vi "Main -simul.vi"() -> ()   [LabVIEW 2013]
uses:
  <vilib>/userdefined/High Color/IMAQdx.ctl
  <vilib>/DAQmx/read.llb/DAQmx Read (Analog 1D Wfm NChan NSamp).vi
  <vilib>/Analysis/baseanly.llb/Mean (DBL).vi
  <vilib>/DAQmx/miscellaneous.llb/DAQmx Fill In Error Info.vi
  <vilib>/measure/madcrms.llb/Basic Averaged DC-RMS for 1 Chan.vi
  <vilib>/measure/mascope.llb/Amplitude and Levels 1 chan.vi
  <vilib>/measure/mamon.llb/Trigger Detection for 1 Channel.vi
  <vilib>/Waveform/WDTOps.llb/WDT Append Waveforms DBL.vi
  <vilib>/measure/NI_MAPro.lvlib
  <vilib>/Analysis/NI_AALBase.lvlib
  <vilib>/vision/driver/NI_Vision_Acquisition_Software.lvlib
panel:
  out "dt":u32
  in  "탭 컨트롤":T1(tab)
  out "웨이브폼 차트 2":dbl(graph)
  in  "reset":bool
  out "right":dbl(slide) scale=0.0..0.5
  out "left":dbl(slide)
  out "rear":dbl(slide) scale=0.0..0.5
  out "front":dbl(slide)
  out "trigger":bool
  in  "Force cal val":bool
  out "Triggered Force graph":waveform(dbl)(graph)={"t0"=timestamp(0 s since 1904-01-01), "dt"=0.00062, "Y"=array[3100 elements]}
  out "bonding force":dbl=1.1386680148675508 caption="Bonding force (kg)" format="%.3f"
  out "Bondtime":dbl=0.5053000000000001 caption="Bonding time" format="%.3f"
  out "vacum":dbl=1.2177873383633695 format="%#_3f"
  out "Heater temp":dbl=nan format="%0.2f"
  out "XY 그래프":cluster{dbl[], dbl[]}(graph)
  out "크기 2":i32[](array[numeric])
  out "triiger":bool
  out "숫자형":i32
  in  "simul":bool
  out "vaccum 차트 3":waveform(dbl)(graph)={"t0"=timestamp(3477442777.176875 s since 1904-01-01), "dt"=0.01, "Y"=[0.9261417940939543, 0.9261417940939543, 0.9261417940939543, 0.9261417940939543, 0.9261417940939543, 0.9261417940939543, 0.9261417940939543, 0.9261417940939543, 0.9261417940939543, 0.9261417940939543], "attributes"=variant("NI_ChannelName"=variant(string "전압"), "NI_UnitDescription"=variant(string "Volts"))}
  out "Force raw chart":waveform(dbl)[](graph)=[{"t0"=timestamp(3477442777.13187 s since 1904-01-01), "dt"=0.00062, "Y"=[-1.6112136636470233e-05, -8.569886798010926e-06, -1.9875060209823524e-07, 2.38297423695265e-06, -2.5658168581669667e-06, -1.772821098699811e-06, -4.127955201515539e-06, 6.359857628775875e-07, 4.928880013384412e-07, -3.030881455329775e-06, -1.6476111269731543e-06, -3.5257574105908386e-06, 3.9272455815972755e-06, 4.1657435117466915e-06, 1.9357923056845556e-06, -8.873963893666015e-06, -7.478785108954976e-06, 2.961286460921625e-07, 1.4110617831093333e-07, -1.8980310390713461e-06, 1.6734457588159683e-06, -1.091306434532689e-05, -1.0513727362142483e-06, -6.190924313818898e-06, -1.2540761368932031e-05, -2.1656959207560037e-05, -7.4907097304474685e-06, -3.2872630354662113e-06, -7.950263527933837e-08, -5.964355867846931e-06, -2.4107952296524134e-06, -3.7881010918357573e-06, 2.609546568115507e-06, 1.715182700246618e-06, -5.290612250873919e-06, -6.512889823589868e-06, -3.120361442334684e-07, 5.578846081749961e-06, 7.045614998740958e-06, -1.4627773018794912e-06, -7.937882831116044e-06, -2.595628704294203e-06, 1.2799261966089874e-06, 3.3190306855961753e-07, -3.4363220332503078e-06, -9.953137975658443e-06, 2.3591245238553327e-06, -1.0871470597100204e-06, 8.685197127258367e-07, -7.478785108954976e-06, -8.659321257106097e-06, -4.879210834785539e-06, -3.710590473067321e-06, -4.771888670569855e-06, -1.2516912366543758e-05, -5.576804340679935e-06, -6.274396873296863e-06, -8.546139112344271e-07, 2.2696881098723825e-06, -3.585380986597095e-06, -7.890184386099151e-06, 4.034519211733817e-07, 2.055040781583931e-06, 3.3071514956147953e-06, -2.7625750097582926e-06, -6.900440625190667e-06, 4.2909549706155075e-06, 9.830102788370948e-06, 3.032879356729265e-06, 4.088231671969834e-06, -9.488079817087242e-06, -5.111742111559042e-06, 2.567809552028929e-06, -4.688415860253707e-06, -1.833603522524735e-05, -9.50012139076079e-07, 3.3250388142463035e-06, -2.6135158111173114e-06, -6.769269618278701e-06, -2.0929577385222132e-05, -7.305878065355784e-06, -1.8562943957647073e-06, -3.090505090348801e-06, -3.5257574105908386e-06, -4.932871908254762e-06, -1.033522309183479e-07, -4.169691655199052e-06, 1.94771715199473e-06, -5.254838228130094e-06, -5.147516144541169e-06, 1.2978134427175586e-06, 9.126526251121246e-06, 1.5422725370008507e-06, -4.688415860253707e-06, -2.005353820147982e-06, 4.4518875659287035e-07, 1.7688444872052448e-06, -1.1229213806461855e-06, -6.51885214588969e-06, -1.4490413466475015e-05], "attributes"=variant("NI_ChannelName"=variant(string "변형률_0"), "NI_UnitDescription"=variant(string "Strain"))}, {"t0"=timestamp(3477442777.13187 s since 1904-01-01), "dt"=0.00062, "Y"=[-1.5926450874775857e-06, 1.7934307923881257e-06, -2.236473822173629e-06, -4.09045749208906e-06, -3.881810155491518e-06, 1.7218937409129746e-06, 3.9872386740088464e-06, 1.7192680555871353e-07, 2.2286147427125606e-06, -1.3005373326004466e-06, 3.456670124526979e-06, 8.523920832607e-06, 5.322604705970085e-06, 3.104945216654824e-06, 2.639953345335169e-06, 6.449322569493326e-06, 1.898110120282012e-07, -2.9306233811443237e-07, -7.929552945691535e-06, 2.53892933758521e-05, 6.6698972632327115e-06, 5.113953528386892e-06, 2.425341858268832e-06, -5.911320745626876e-07, -2.8385721664852527e-06, 1.0303694376600552e-06, -3.2286931975534613e-07, -4.793896442446842e-06, -2.7789585013682837e-06, -2.254357941858881e-06, 4.482039064584e-06, 3.188405341896096e-06, 2.890333530003795e-06, 1.5370897386411374e-06, 1.3224787249476363e-06, 5.0603003825103886e-06, 4.470116157849115e-06, 2.0378491288205883e-06, 3.087060905915481e-06, 4.237619533343155e-06, 6.22874797305966e-06, 2.4551490037417866e-06, 8.455656909807571e-07, -1.976799849226179e-07, -2.862417630541878e-06, 5.030493081733363e-06, 2.8068734545164028e-06, -7.640124402846258e-07, -2.105323591603382e-06, 2.3750223240719277e-07, 6.884510572159387e-06, -7.878580032793122e-07, -5.163499562134611e-06, -6.391533772034915e-06, -2.6835766223972933e-06, 4.684728522578421e-06, 2.885317683250044e-08, -1.2826531787987904e-06, -2.8206880676963555e-06, 3.7726266086577194e-06, 6.7414350226397595e-06, 3.3195569954219583e-06, 2.017338166964026e-07, 2.7114905281608864e-06, 3.40301715648635e-06, 9.60891530636603e-06, -7.029395011258529e-06, 2.153804825353152e-05, 1.1194680695472973e-05, -9.786224662971449e-07, 8.702765913475292e-06, -2.558387878634849e-06, -5.911320745626876e-07, -2.4272377325028147e-06, 2.8307191889483254e-06, 5.656446771208991e-06, 1.9901577367198323e-06, -2.2960875519699664e-06, -4.656785538247539e-06, -2.898185824494624e-06, 7.501831387741804e-07, -3.983153158427838e-06, -1.610529230191517e-06, -2.8028039682679484e-06, 4.458193251398366e-06, 9.171026170763248e-07, 3.748780829304955e-06, 1.9577241432685033e-07, 3.206289656260379e-06, 2.0974633753433343e-06, 7.442217298655735e-07, 6.548006047634227e-07, -1.8489844052503307e-06, 3.7964723891478954e-06, 8.0470009297029e-06, 2.5863004649327575e-06, 1.1674819390124968e-06, 3.150004752252312e-07, 3.188405341896096e-06, 5.7637531966593845e-06], "attributes"=variant("NI_ChannelName"=variant(string "변형률_1"), "NI_UnitDescription"=variant(string "Strain"))}, {"t0"=timestamp(3477442777.13187 s since 1904-01-01), "dt"=0.00062, "Y"=[-9.774144215970737e-06, -5.761376757146625e-06, 5.947220028941115e-07, -3.8056626676763385e-06, -7.275857412313684e-06, 3.1765375395588494e-06, -3.1557437920494864e-06, -3.000717146469372e-06, 7.974506851273759e-07, -1.8618660842482212e-06, -1.4862235419361472e-06, -6.721343374039278e-06, 8.62045556081355e-06, -3.294812422418737e-07, 2.115189123215763e-06, -2.3030966465335333e-06, -5.773301819593379e-06, -1.1940569250260916e-06, -5.171085810533189e-06, -2.538875015539028e-08, 3.6814298472928053e-07, -8.939395837287375e-06, 2.401395215885246e-06, -4.646382161832467e-06, -7.311632490439199e-06, -2.205074690463858e-05, -3.5313850800753163e-06, -4.425767963291082e-06, -3.6148608835335274e-06, -1.677026138378287e-06, -2.5952626153941553e-06, 3.26404755740087e-07, -2.601225184409818e-06, 1.4056372250135049e-06, -1.1753684800069817e-05, -4.914696596438629e-06, 5.808765257422834e-08, 6.318857576908811e-06, 3.9934195965366175e-06, 5.03688401927312e-06, -6.059503232998047e-06, -5.4811377077647035e-06, 1.3937119916306282e-06, -7.055244373975443e-06, 7.318619848217363e-07, -1.718764196644247e-06, 4.814324809771893e-07, -1.0119968136008337e-05, 1.984011385493666e-06, -1.0131893094502119e-05, -1.0251142663796572e-05, -3.865288210289022e-06, -6.06546576070178e-06, -6.995619211769368e-06, 2.1867406310243084e-06, -1.0119968136008337e-05, -8.080796051007461e-06, -1.7962777241804084e-06, -1.2536827790775241e-06, 1.4771886312832808e-06, 2.2284790153078483e-06, -6.190678826058288e-06, -1.7068390374955085e-06, 1.4593007787556523e-06, 5.024958699283277e-06, 2.1927032571370627e-06, 5.589463616211063e-07, -4.831221009990731e-06, -8.959275481128778e-07, 3.421005752440379e-06, 3.987456948949547e-06, -4.205153667407975e-06, -9.674786147839707e-07, -5.212823577128643e-06, -1.6183772832057885e-05, 9.294241431321112e-06, -3.257107342016943e-06, -4.473468338791205e-06, -1.0316729914785664e-05, -1.128265025116678e-05, -1.0650628513704086e-05, -4.65234470638786e-06, -2.362722368329657e-06, -7.230124280525015e-07, 7.139741589589915e-07, -2.326946936105031e-06, -1.5277486145651072e-05, 1.411599841811428e-06, -3.3703959911923048e-06, -5.7852268817560655e-06, 2.17481537901177e-06, 2.5325730631100896e-06, -1.981117625965015e-06, -2.3209843638189005e-06, -2.6191128910294843e-06, 9.047776678219688e-07, -6.514613263977364e-07, -9.495908490762017e-07, 5.470211484321648e-07, -1.2970025127066287e-05], "attributes"=variant("NI_ChannelName"=variant(string "변형률_2"), "NI_UnitDescription"=variant(string "Strain"))}, {"t0"=timestamp(3477442777.13187 s since 1904-01-01), "dt"=0.00062, "Y"=[-7.598292136517871e-06, -3.990960943167142e-06, -3.961148180242939e-06, 8.446924425047726e-07, -3.865747326939833e-06, -6.459578537381319e-07, -5.028556181360945e-07, -4.313044849763774e-07, -2.0352399287900154e-06, -2.1843042998043006e-06, 2.317459299605134e-06, 2.520188680335006e-06, 1.8642998046072807e-06, 3.1998303138911986e-07, -2.3810692014959805e-06, 1.1129194138591358e-07, -3.919410309162601e-06, -4.181762583788524e-06, -2.9177003579997263e-06, -2.887887531081505e-06, 8.147893563887326e-08, -5.910899132064934e-06, 5.841384650575335e-06, -7.771348670609545e-07, -9.965402760758176e-06, -5.064219224553743e-06, -1.0078689889986319e-05, -8.14684269941332e-06, -4.8913055460130025e-06, -2.0292773530250545e-06, -2.5003206193811262e-06, -4.098286874975869e-06, -3.305266946174274e-06, -4.038661360148547e-06, -2.4228072009909966e-06, -2.1366037059148034e-06, -4.217537883299131e-06, -1.2183663865814867e-06, -2.5062831895288145e-06, 1.1725454274867201e-07, 3.9571845882479464e-06, -1.8087543828407676e-07, -4.0803992212742764e-06, -1.2064412154978175e-06, -5.839348772806825e-06, -1.8563626249113895e-06, -5.213282692541838e-06, -3.1800531582297593e-06, -1.8742503581789873e-06, -3.8360372384809986e-07, -4.181762583788524e-06, -6.0420747641119605e-06, -4.050586463682811e-06, -3.531844197032469e-06, -2.3452937705841765e-06, -7.1034036122986465e-06, -1.32569291353597e-06, -1.6953729967054738e-06, -1.7549987909737935e-06, -2.8699998340773e-06, -4.825717583337447e-06, -2.46454519700197e-06, 1.1964865605783791e-06, 3.378708431566748e-07, 2.889871880335409e-06, 2.0908795007679327e-06, -1.0514139655274806e-06, 5.501512595474361e-06, -3.376817668063878e-06, -4.819755040849376e-06, -1.5701588055974375e-06, -5.064219224553743e-06, -8.904240781442745e-07, 4.028736359651292e-06, -4.1996502338637966e-06, -6.918565604118794e-06, -3.996923495538705e-06, -3.3648925484600175e-06, -1.3024146240405366e-05, -8.289942747279497e-06, -7.061666003521132e-06, -5.165582387620764e-06, -6.823165315097408e-06, -1.0633391403086943e-06, -1.9517638616103747e-06, -5.255020455614867e-06, -2.4705077675762867e-06, -1.7491284040547266e-07, -3.1919782822420984e-06, -2.858074702385669e-06, -1.9815767443457687e-06, 2.317459299605134e-06, 3.927371353185168e-06, 3.665014961285459e-06, 2.186281508816372e-06, -1.0096758515535991e-06, -1.5522710614508004e-06, -6.507151727700881e-06, -2.16045400342839e-06, -2.893850096607393e-06], "attributes"=variant("NI_ChannelName"=variant(string "변형률_3"), "NI_UnitDescription"=variant(string "Strain"))}]
  in  "display":bool=TRUE
  out "vacum 2":dbl=0.9261417940939543 format="%#_3f"
  out "x-y 2":u32=56
  out "x-y":u32=99
  out "Filtered force 차트":waveform(dbl)[](graph)
  out "Force raw graph":waveform(dbl)[](graph)=[{"t0"=timestamp(3477442777.13187 s since 1904-01-01), "dt"=0.00062, "Y"=[-1.6112136636470233e-05, -8.569886798010926e-06, -1.9875060209823524e-07, 2.38297423695265e-06, -2.5658168581669667e-06, -1.772821098699811e-06, -4.127955201515539e-06, 6.359857628775875e-07, 4.928880013384412e-07, -3.030881455329775e-06, -1.6476111269731543e-06, -3.5257574105908386e-06, 3.9272455815972755e-06, 4.1657435117466915e-06, 1.9357923056845556e-06, -8.873963893666015e-06, -7.478785108954976e-06, 2.961286460921625e-07, 1.4110617831093333e-07, -1.8980310390713461e-06, 1.6734457588159683e-06, -1.091306434532689e-05, -1.0513727362142483e-06, -6.190924313818898e-06, -1.2540761368932031e-05, -2.1656959207560037e-05, -7.4907097304474685e-06, -3.2872630354662113e-06, -7.950263527933837e-08, -5.964355867846931e-06, -2.4107952296524134e-06, -3.7881010918357573e-06, 2.609546568115507e-06, 1.715182700246618e-06, -5.290612250873919e-06, -6.512889823589868e-06, -3.120361442334684e-07, 5.578846081749961e-06, 7.045614998740958e-06, -1.4627773018794912e-06, -7.937882831116044e-06, -2.595628704294203e-06, 1.2799261966089874e-06, 3.3190306855961753e-07, -3.4363220332503078e-06, -9.953137975658443e-06, 2.3591245238553327e-06, -1.0871470597100204e-06, 8.685197127258367e-07, -7.478785108954976e-06, -8.659321257106097e-06, -4.879210834785539e-06, -3.710590473067321e-06, -4.771888670569855e-06, -1.2516912366543758e-05, -5.576804340679935e-06, -6.274396873296863e-06, -8.546139112344271e-07, 2.2696881098723825e-06, -3.585380986597095e-06, -7.890184386099151e-06, 4.034519211733817e-07, 2.055040781583931e-06, 3.3071514956147953e-06, -2.7625750097582926e-06, -6.900440625190667e-06, 4.2909549706155075e-06, 9.830102788370948e-06, 3.032879356729265e-06, 4.088231671969834e-06, -9.488079817087242e-06, -5.111742111559042e-06, 2.567809552028929e-06, -4.688415860253707e-06, -1.833603522524735e-05, -9.50012139076079e-07, 3.3250388142463035e-06, -2.6135158111173114e-06, -6.769269618278701e-06, -2.0929577385222132e-05, -7.305878065355784e-06, -1.8562943957647073e-06, -3.090505090348801e-06, -3.5257574105908386e-06, -4.932871908254762e-06, -1.033522309183479e-07, -4.169691655199052e-06, 1.94771715199473e-06, -5.254838228130094e-06, -5.147516144541169e-06, 1.2978134427175586e-06, 9.126526251121246e-06, 1.5422725370008507e-06, -4.688415860253707e-06, -2.005353820147982e-06, 4.4518875659287035e-07, 1.7688444872052448e-06, -1.1229213806461855e-06, -6.51885214588969e-06, -1.4490413466475015e-05], "attributes"=variant("NI_ChannelName"=variant(string "변형률_0"), "NI_UnitDescription"=variant(string "Strain"))}, {"t0"=timestamp(3477442777.13187 s since 1904-01-01), "dt"=0.00062, "Y"=[-1.5926450874775857e-06, 1.7934307923881257e-06, -2.236473822173629e-06, -4.09045749208906e-06, -3.881810155491518e-06, 1.7218937409129746e-06, 3.9872386740088464e-06, 1.7192680555871353e-07, 2.2286147427125606e-06, -1.3005373326004466e-06, 3.456670124526979e-06, 8.523920832607e-06, 5.322604705970085e-06, 3.104945216654824e-06, 2.639953345335169e-06, 6.449322569493326e-06, 1.898110120282012e-07, -2.9306233811443237e-07, -7.929552945691535e-06, 2.53892933758521e-05, 6.6698972632327115e-06, 5.113953528386892e-06, 2.425341858268832e-06, -5.911320745626876e-07, -2.8385721664852527e-06, 1.0303694376600552e-06, -3.2286931975534613e-07, -4.793896442446842e-06, -2.7789585013682837e-06, -2.254357941858881e-06, 4.482039064584e-06, 3.188405341896096e-06, 2.890333530003795e-06, 1.5370897386411374e-06, 1.3224787249476363e-06, 5.0603003825103886e-06, 4.470116157849115e-06, 2.0378491288205883e-06, 3.087060905915481e-06, 4.237619533343155e-06, 6.22874797305966e-06, 2.4551490037417866e-06, 8.455656909807571e-07, -1.976799849226179e-07, -2.862417630541878e-06, 5.030493081733363e-06, 2.8068734545164028e-06, -7.640124402846258e-07, -2.105323591603382e-06, 2.3750223240719277e-07, 6.884510572159387e-06, -7.878580032793122e-07, -5.163499562134611e-06, -6.391533772034915e-06, -2.6835766223972933e-06, 4.684728522578421e-06, 2.885317683250044e-08, -1.2826531787987904e-06, -2.8206880676963555e-06, 3.7726266086577194e-06, 6.7414350226397595e-06, 3.3195569954219583e-06, 2.017338166964026e-07, 2.7114905281608864e-06, 3.40301715648635e-06, 9.60891530636603e-06, -7.029395011258529e-06, 2.153804825353152e-05, 1.1194680695472973e-05, -9.786224662971449e-07, 8.702765913475292e-06, -2.558387878634849e-06, -5.911320745626876e-07, -2.4272377325028147e-06, 2.8307191889483254e-06, 5.656446771208991e-06, 1.9901577367198323e-06, -2.2960875519699664e-06, -4.656785538247539e-06, -2.898185824494624e-06, 7.501831387741804e-07, -3.983153158427838e-06, -1.610529230191517e-06, -2.8028039682679484e-06, 4.458193251398366e-06, 9.171026170763248e-07, 3.748780829304955e-06, 1.9577241432685033e-07, 3.206289656260379e-06, 2.0974633753433343e-06, 7.442217298655735e-07, 6.548006047634227e-07, -1.8489844052503307e-06, 3.7964723891478954e-06, 8.0470009297029e-06, 2.5863004649327575e-06, 1.1674819390124968e-06, 3.150004752252312e-07, 3.188405341896096e-06, 5.7637531966593845e-06], "attributes"=variant("NI_ChannelName"=variant(string "변형률_1"), "NI_UnitDescription"=variant(string "Strain"))}, {"t0"=timestamp(3477442777.13187 s since 1904-01-01), "dt"=0.00062, "Y"=[-9.774144215970737e-06, -5.761376757146625e-06, 5.947220028941115e-07, -3.8056626676763385e-06, -7.275857412313684e-06, 3.1765375395588494e-06, -3.1557437920494864e-06, -3.000717146469372e-06, 7.974506851273759e-07, -1.8618660842482212e-06, -1.4862235419361472e-06, -6.721343374039278e-06, 8.62045556081355e-06, -3.294812422418737e-07, 2.115189123215763e-06, -2.3030966465335333e-06, -5.773301819593379e-06, -1.1940569250260916e-06, -5.171085810533189e-06, -2.538875015539028e-08, 3.6814298472928053e-07, -8.939395837287375e-06, 2.401395215885246e-06, -4.646382161832467e-06, -7.311632490439199e-06, -2.205074690463858e-05, -3.5313850800753163e-06, -4.425767963291082e-06, -3.6148608835335274e-06, -1.677026138378287e-06, -2.5952626153941553e-06, 3.26404755740087e-07, -2.601225184409818e-06, 1.4056372250135049e-06, -1.1753684800069817e-05, -4.914696596438629e-06, 5.808765257422834e-08, 6.318857576908811e-06, 3.9934195965366175e-06, 5.03688401927312e-06, -6.059503232998047e-06, -5.4811377077647035e-06, 1.3937119916306282e-06, -7.055244373975443e-06, 7.318619848217363e-07, -1.718764196644247e-06, 4.814324809771893e-07, -1.0119968136008337e-05, 1.984011385493666e-06, -1.0131893094502119e-05, -1.0251142663796572e-05, -3.865288210289022e-06, -6.06546576070178e-06, -6.995619211769368e-06, 2.1867406310243084e-06, -1.0119968136008337e-05, -8.080796051007461e-06, -1.7962777241804084e-06, -1.2536827790775241e-06, 1.4771886312832808e-06, 2.2284790153078483e-06, -6.190678826058288e-06, -1.7068390374955085e-06, 1.4593007787556523e-06, 5.024958699283277e-06, 2.1927032571370627e-06, 5.589463616211063e-07, -4.831221009990731e-06, -8.959275481128778e-07, 3.421005752440379e-06, 3.987456948949547e-06, -4.205153667407975e-06, -9.674786147839707e-07, -5.212823577128643e-06, -1.6183772832057885e-05, 9.294241431321112e-06, -3.257107342016943e-06, -4.473468338791205e-06, -1.0316729914785664e-05, -1.128265025116678e-05, -1.0650628513704086e-05, -4.65234470638786e-06, -2.362722368329657e-06, -7.230124280525015e-07, 7.139741589589915e-07, -2.326946936105031e-06, -1.5277486145651072e-05, 1.411599841811428e-06, -3.3703959911923048e-06, -5.7852268817560655e-06, 2.17481537901177e-06, 2.5325730631100896e-06, -1.981117625965015e-06, -2.3209843638189005e-06, -2.6191128910294843e-06, 9.047776678219688e-07, -6.514613263977364e-07, -9.495908490762017e-07, 5.470211484321648e-07, -1.2970025127066287e-05], "attributes"=variant("NI_ChannelName"=variant(string "변형률_2"), "NI_UnitDescription"=variant(string "Strain"))}, {"t0"=timestamp(3477442777.13187 s since 1904-01-01), "dt"=0.00062, "Y"=[-7.598292136517871e-06, -3.990960943167142e-06, -3.961148180242939e-06, 8.446924425047726e-07, -3.865747326939833e-06, -6.459578537381319e-07, -5.028556181360945e-07, -4.313044849763774e-07, -2.0352399287900154e-06, -2.1843042998043006e-06, 2.317459299605134e-06, 2.520188680335006e-06, 1.8642998046072807e-06, 3.1998303138911986e-07, -2.3810692014959805e-06, 1.1129194138591358e-07, -3.919410309162601e-06, -4.181762583788524e-06, -2.9177003579997263e-06, -2.887887531081505e-06, 8.147893563887326e-08, -5.910899132064934e-06, 5.841384650575335e-06, -7.771348670609545e-07, -9.965402760758176e-06, -5.064219224553743e-06, -1.0078689889986319e-05, -8.14684269941332e-06, -4.8913055460130025e-06, -2.0292773530250545e-06, -2.5003206193811262e-06, -4.098286874975869e-06, -3.305266946174274e-06, -4.038661360148547e-06, -2.4228072009909966e-06, -2.1366037059148034e-06, -4.217537883299131e-06, -1.2183663865814867e-06, -2.5062831895288145e-06, 1.1725454274867201e-07, 3.9571845882479464e-06, -1.8087543828407676e-07, -4.0803992212742764e-06, -1.2064412154978175e-06, -5.839348772806825e-06, -1.8563626249113895e-06, -5.213282692541838e-06, -3.1800531582297593e-06, -1.8742503581789873e-06, -3.8360372384809986e-07, -4.181762583788524e-06, -6.0420747641119605e-06, -4.050586463682811e-06, -3.531844197032469e-06, -2.3452937705841765e-06, -7.1034036122986465e-06, -1.32569291353597e-06, -1.6953729967054738e-06, -1.7549987909737935e-06, -2.8699998340773e-06, -4.825717583337447e-06, -2.46454519700197e-06, 1.1964865605783791e-06, 3.378708431566748e-07, 2.889871880335409e-06, 2.0908795007679327e-06, -1.0514139655274806e-06, 5.501512595474361e-06, -3.376817668063878e-06, -4.819755040849376e-06, -1.5701588055974375e-06, -5.064219224553743e-06, -8.904240781442745e-07, 4.028736359651292e-06, -4.1996502338637966e-06, -6.918565604118794e-06, -3.996923495538705e-06, -3.3648925484600175e-06, -1.3024146240405366e-05, -8.289942747279497e-06, -7.061666003521132e-06, -5.165582387620764e-06, -6.823165315097408e-06, -1.0633391403086943e-06, -1.9517638616103747e-06, -5.255020455614867e-06, -2.4705077675762867e-06, -1.7491284040547266e-07, -3.1919782822420984e-06, -2.858074702385669e-06, -1.9815767443457687e-06, 2.317459299605134e-06, 3.927371353185168e-06, 3.665014961285459e-06, 2.186281508816372e-06, -1.0096758515535991e-06, -1.5522710614508004e-06, -6.507151727700881e-06, -2.16045400342839e-06, -2.893850096607393e-06], "attributes"=variant("NI_ChannelName"=variant(string "변형률_3"), "NI_UnitDescription"=variant(string "Strain"))}]
  out "Filtered force 그래프":waveform(dbl)[](graph)
  out "Strain front":dbl(graph)=0.21080623907694704
  out "Strain left":dbl(graph)=0.40238302318753916
  out "Strain rear":dbl(graph)=0.4140902820131476
  out "Strain right":dbl(graph)=0.09497703213784708
  out "강도 그래프 2":dbl[][](graph)=[[nan, nan, nan, nan], [nan, nan, nan, nan]]
  out "Image":T2(plugin-control)
  out "error out":errorcluster={"status"=FALSE, "code"=-1074360308, "source"=""}
  out "Heater temp 2":dbl=nan caption="Heater temp" format="%0.2f"
  out "웨이브폼 차트":u32(graph)
  out "data":dynamicdata(graph)=[{"t0"=timestamp(3477442777.176875 s since 1904-01-01), "dt"=0.01, "Y"=[0.9261417940939543, 0.9261417940939543, 0.9261417940939543, 0.9261417940939543, 0.9261417940939543, 0.9261417940939543, 0.9261417940939543, 0.9261417940939543, 0.9261417940939543, 0.9261417940939543], "attributes"=variant("NI_ChannelName"=variant(string "전압"), "NI_UnitDescription"=variant(string "Volts"))}] caption="데이터"
  in  "bonding time trigger edge level":dbl=0.5 format="%#_13g"
  out "front mean":dbl=0.24100886710135544 format="%0.2f"
  out "left mean":dbl=0.5329196805184643 format="%0.2f"
  out "rear mean 3":dbl=0.3563222576715275 caption="rear mean" format="%0.2f"
  out "right mean 4":dbl=0.1826222935697912 caption="right mean" format="%0.2f"
  in  "Force trigger minimum level":dbl=0.5 format="%#_13g"
  in  "state settings":T3={"method"=enum."histogram", "histogram size"=512, "histogram method"=enum."mode", "reserved"=1.0} caption="상태 셋팅" {"reserved" format="%0.2f"}
  out "level1 4":dbl=0.09497703213784708 caption="right F" format="%.2g"
  out "level1 3":dbl=0.4140902820131476 caption="rear F" format="%.2g"
  out "level1 2":dbl=0.40238302318753916 caption="left F" format="%.2g"
  out "level1":dbl=0.21080623907694704 caption="front F" format="%.2g"
  in  "Lower Cut-Off":dbl=20.0 caption="하위 컷오프"
  out "웨이브폼 그래프 2":waveform(dbl)(graph)
  out "웨이브폼 그래프":waveform(dbl)(graph)
  out "force offset":dbl
  out "trigger location 2":dbl=1.84016 caption="트리거 falling" format="%#.3f"
  out "trigger location":dbl=1.33486 caption="트리거 rising" format="%#.3f"
  out "strain high level mean":T4={"mean"=0.24100886710135544, "mean"=0.5329196805184643, "mean"=0.3563222576715275, "mean"=0.1826222935697912}
  in  "정지":bool=TRUE
  # "Die Attach Machine Monitoring"
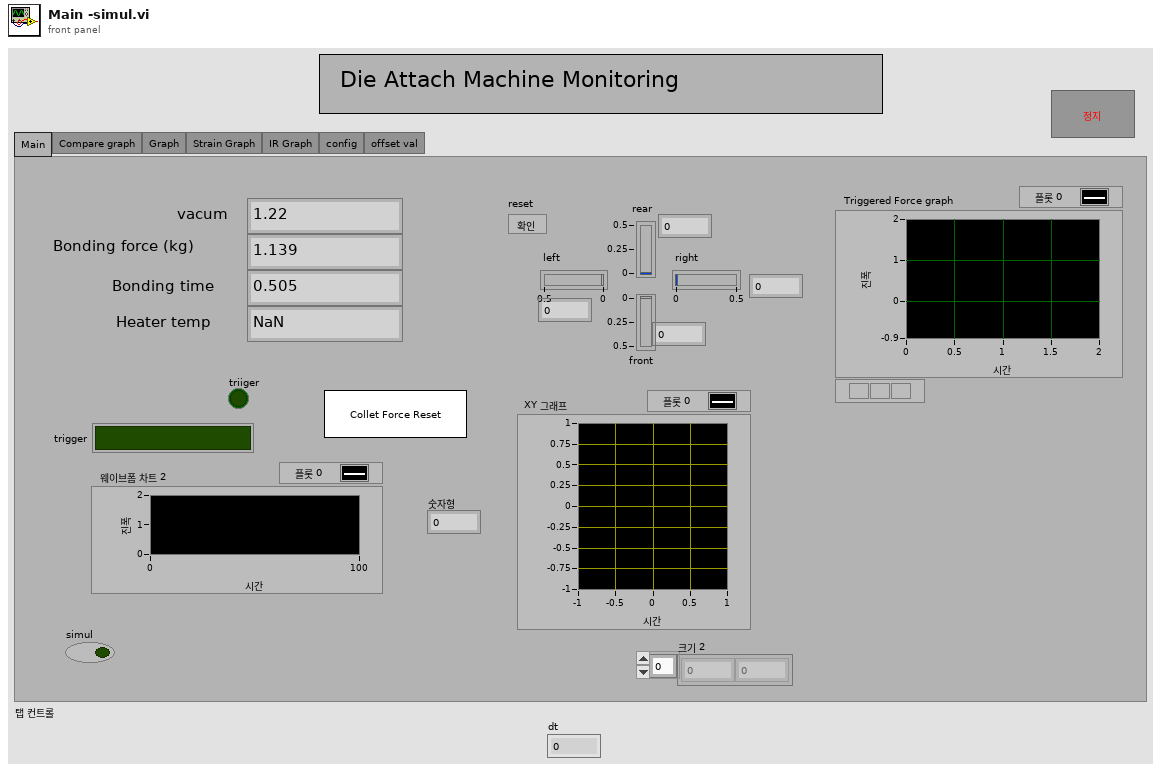
[diagram p1: front panel]
types:
  T1 = enum32{"Main", "Compare graph", "Graph", "Strain Graph", "IR Graph", "config", "offset val"}
  T2 = typedef "IMAQ Image.ctl" = refnum<image>
  T3 = cluster{"method":enum32{"histogram", "peak", "auto select"}, "histogram size":i32, "histogram method":enum16{"mode"}, "reserved":dbl}
  T4 = cluster{"mean":dbl, "mean":dbl, "mean":dbl, "mean":dbl}
  T5 = typedef "IMAQdx.ctl" = refnum<k21>
  T6 = cluster{"Global Rectangle":i32[], "Contours":cluster{"Contour Type":u32, "ROI Type":u32, "Points":i32[]}[]}
  T7 = cluster{"high state level":dbl, "high state level":dbl, "high state level":dbl, "high state level":dbl}
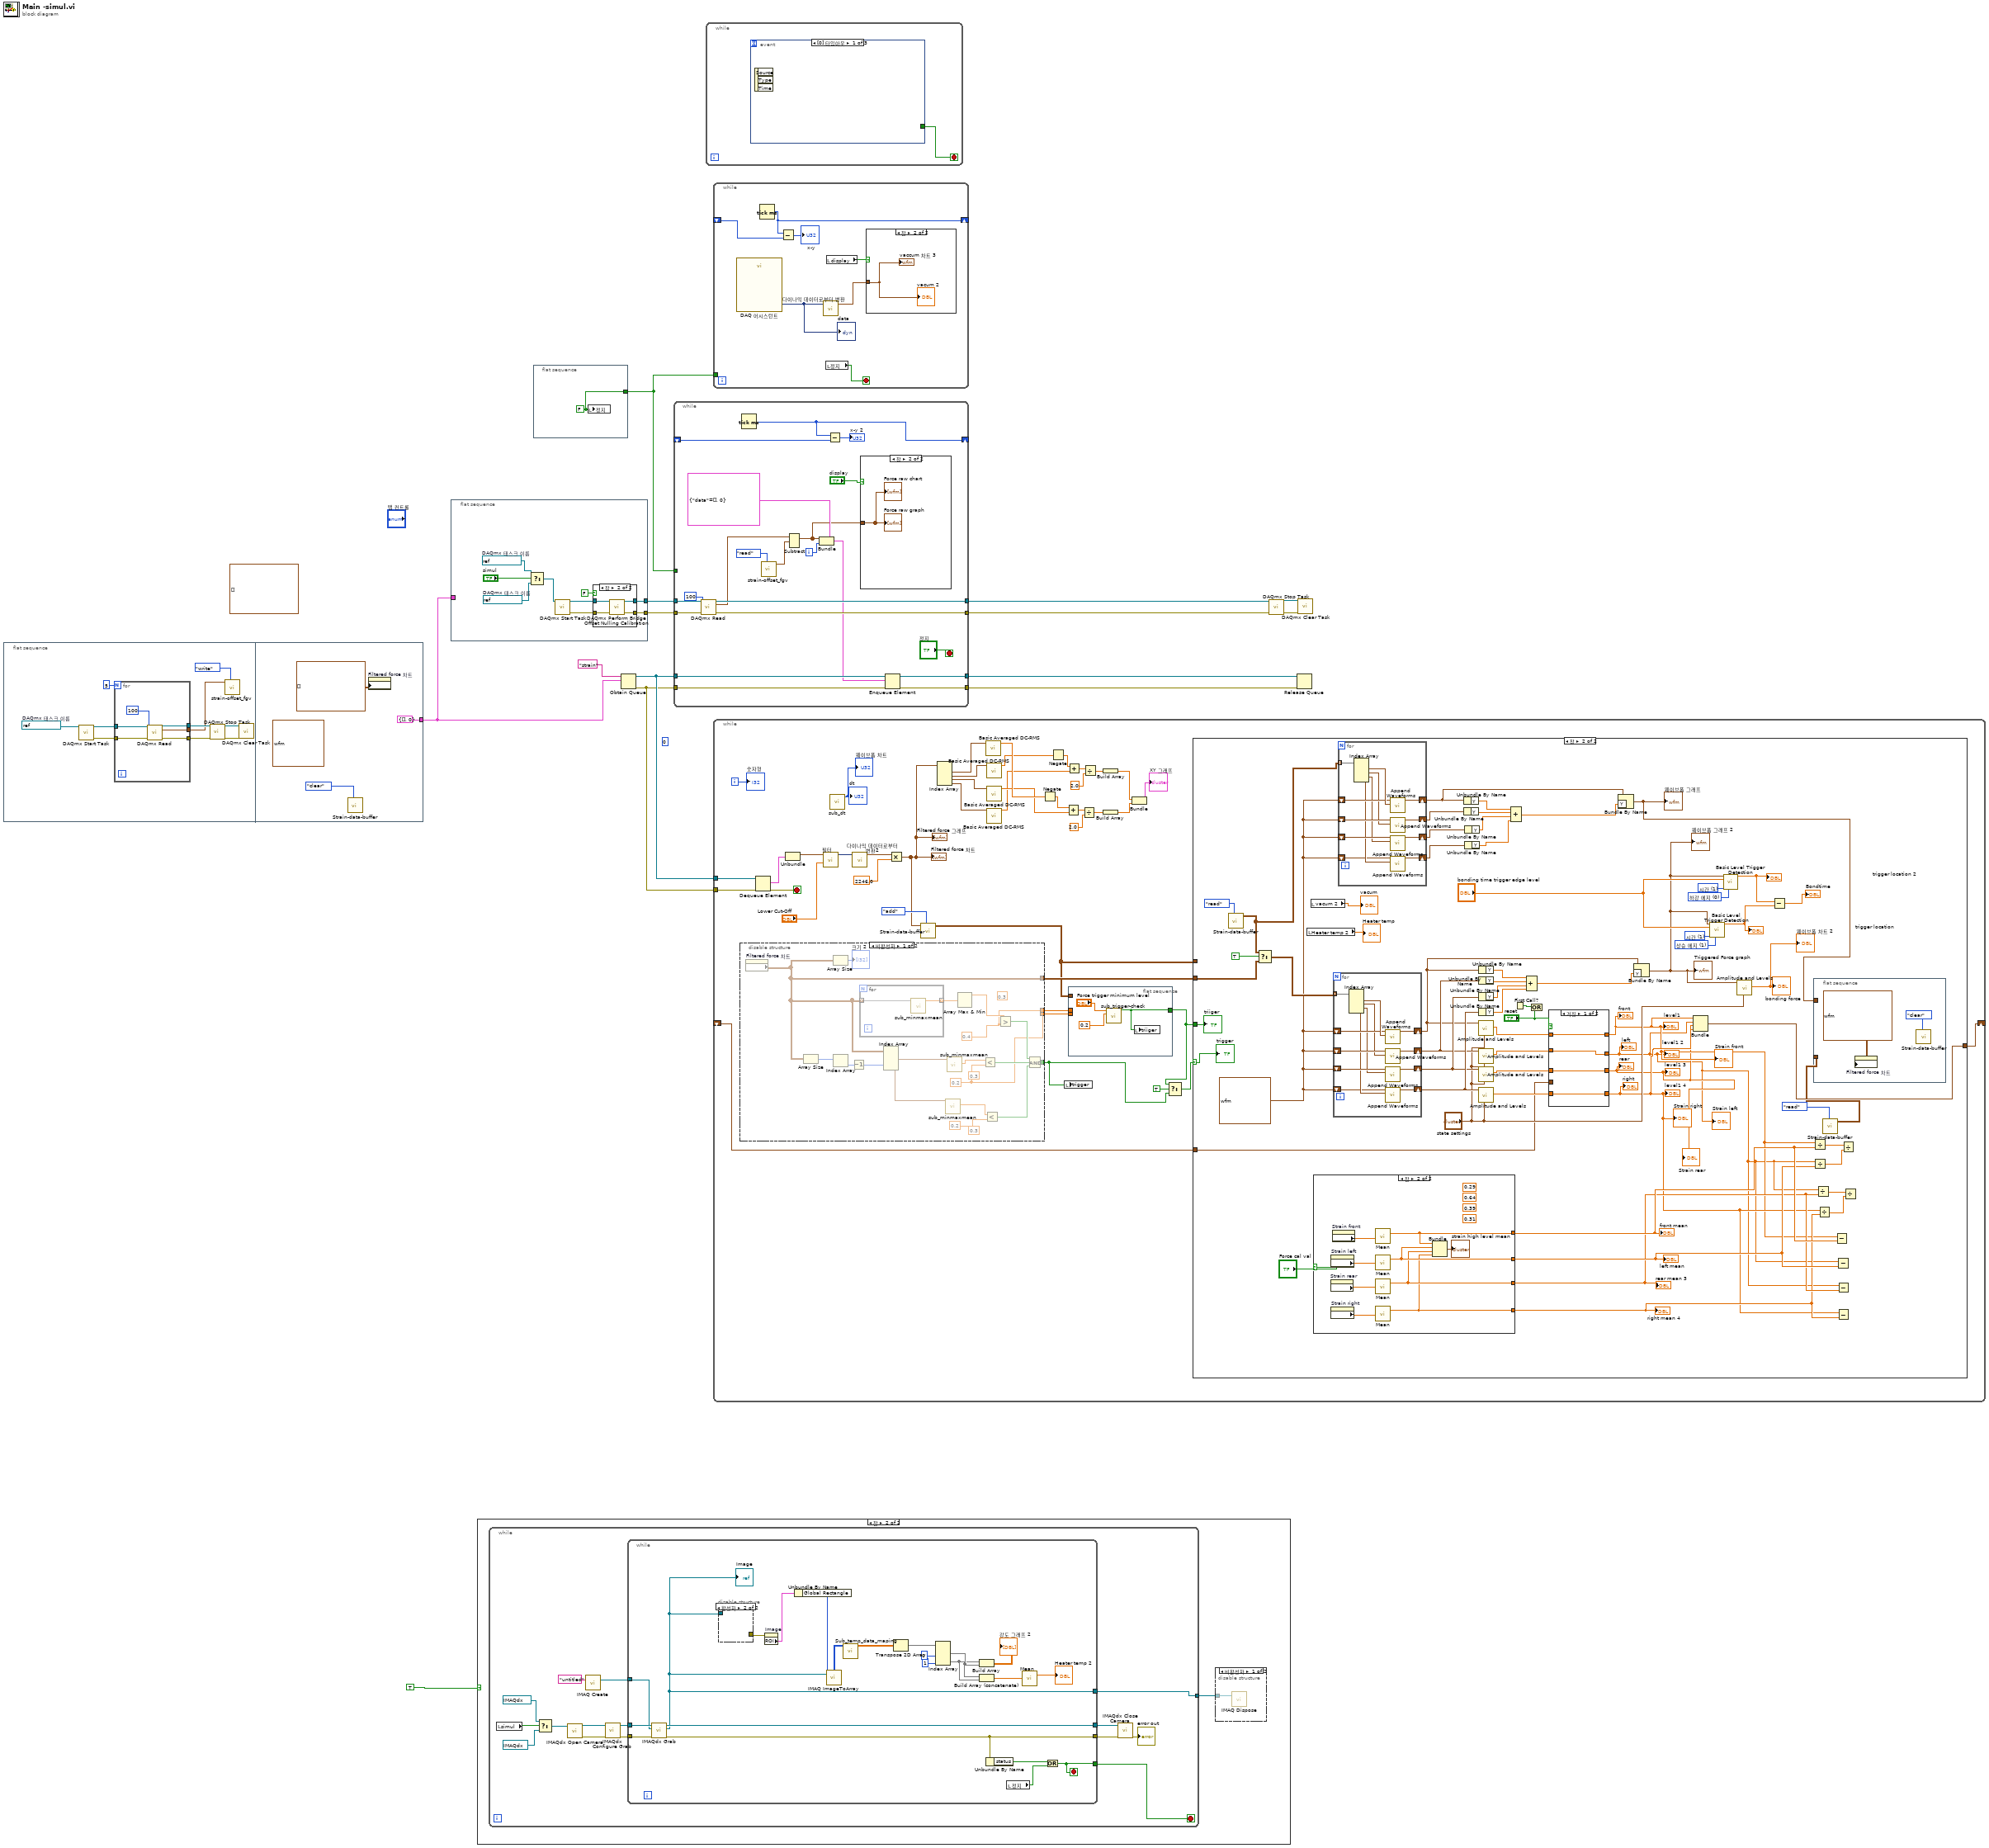
[diagram p0: block diagram]
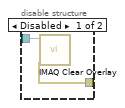
[diagram p4: hidden frame]
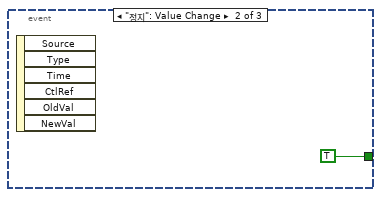
[diagram p6: hidden frame]
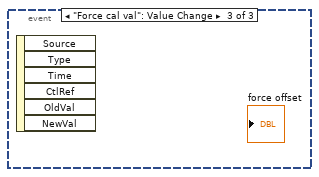
[diagram p7: hidden frame]
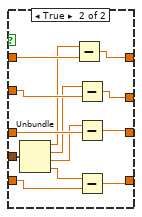
[diagram p10: hidden frame]
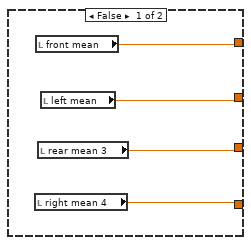
[diagram p11: hidden frame]
diagram:
  (unwired) waveform(dbl)[] [] ("data")
  (unwired) 0 ("y")
  n1 = flat-sequence {
    tunnel: [cluster{"data":waveform(dbl)[], i32} {"data"=[], 0}] -> w1
    frame #0 {
      w24 = refnum<k21> "9237_task"  # DAQmx 태스크 이름
      n2 = call <vilib>:"DAQmx Start Task.vi"("task/channels in"=w24) -> ("task out"=w22:refnum<k21>, "error out"=w23:errorcluster)  [unwired: 13 in]
      n3 = for {
        N: 5 -> [_]
        tunnel: w23 -> [w29]
        tunnel: w22 -> [w28]
        tunnel: [w27] -> w19
        tunnel: [w26] -> w18
        tunnel: [w25] -> w16
        n4 = call-poly <vilib>:"DAQmx Read.vi"("task/channels in"=w28, "number of samples per channel"=100, "error in"=w29) -> ("task out"=w26:refnum<k21>, "data"=w25:waveform(dbl)[], "error out"=w27:errorcluster)  [unwired: 10 in]
      }
      n5 = call <vilib>:"DAQmx Stop Task.vi"("task/channels in"=w18, "error in"=w19) -> ("task out"=w20:refnum<k21>, "error out"=w21:errorcluster)  [unwired: 12 in]
      n6 = call "strain-offset_fgv.vi"("열거형"=enum16{"write", "read"}."write", "data"=w16) -> ()  [unwired: 9 in, 1 out]
      n7 = call <vilib>:"DAQmx Clear Task.vi"("task in"=w20, "error in"=w21) -> ()  [unwired: 13 in, 1 out]
    }
    frame #1 {
      (unwired) waveform(dbl) {"t0"=timestamp(0 s since 1904-01-01), "dt"=1.0, "Y"=[]} ("Waveform")
      n8 = call "Strain-data-buffer.vi"("cmd"=enum16{"clear", "add", "read"}."clear") -> ()  [unwired: 10 in, 1 out]
      n9 = property on="Filtered force 차트" class="WFChart (엄격한)"("History Data"=waveform(dbl)[][] [] ("히스토리 데이터")) -> ()  [unwired: 2 in, 2 out]
    }
  }
  n10 = flat-sequence {
    tunnel: [w40] -> w4
    tunnel: [w39] -> w3
    tunnel: w1 -> [_]
    frame #0 {
      w36 = refnum<k21> "9237_task"  # DAQmx 태스크 이름
      w37 = refnum<k21> "9237_task"  # DAQmx 태스크 이름
      n11 = Select(t=w36, s="simul", f=w37) -> (s? t:f=w34:refnum<k21>)
      n12 = call <vilib>:"DAQmx Start Task.vi"("task/channels in"=w34) -> ("task out"=w42:refnum<k21>, "error out"=w41:errorcluster)  [unwired: 13 in]
      n13 = case shown="참" FALSE {
        tunnel: w42 -> [w44 w48]
        tunnel: w41 -> [w43 w47]
        tunnel: [w43 w46] -> w40
        tunnel: [w44 w45] -> w39
        frame False {
        }
        frame True {
          n14 = call <vilib>:"DAQmx Perform Bridge Offset Nulling Calibration.vi"("task/channels in"=w48, "error in"=w47) -> ("task out"=w45:refnum<k21>, "error out"=w46:errorcluster)  [unwired: 12 in]
        }
      }
    }
  }
  n15 = case shown="참" TRUE {
    frame False {
    }
    frame True {
      n16 = while {
        tunnel: [w56] -> w49
        stop <- w55 stop-if-true
        n17 = local read "simul"() -> (w50:bool)
        n18 = Select(t=T5 "cam0" ("Session In"), s=w50, f=T5 "ssw" ("Session In")) -> (s? t:f=w51:T5)
        n19 = call <vilib>:"IMAQdx Open Camera.vi"("Session In"=w51) -> ("error out"=w61:errorcluster, "Session Out"=w64:T5)  [unwired: 9 in]
        n20 = call "IMAQ Create"("Image Name"="untitled") -> ("New Image"=w58:T2)  [unwired: 4 in, 1 out]
        n21 = call <vilib>:"IMAQdx Configure Grab.vi"("error in"=w61, "Session In"=w64) -> ("error out"=w60:errorcluster, "Session Out"=w63:T5)  [unwired: 8 in]
        n22 = while {
          tunnel: w63 -> [w86]
          tunnel: [w85] -> w62
          tunnel: w60 -> [w84]
          tunnel: [w82] -> w59
          tunnel: w58 -> [w83]
          tunnel: [w71] -> w56
          tunnel: [w66] -> w55
          stop <- w66 stop-if-true
          n23 = call <vilib>:"IMAQdx Grab.vi"("error in"=w84, "Image In"=w83, "Session In"=w86) -> ("error out"=w82:errorcluster, "Image Out"=w71:T2, "Session Out"=w85:T5)  [unwired: 5 in, 1 out]
          "Image" <- w71
          n24 = disable-structure shown="활성화" {
            disable-tunnel: w71 -> [w88 _]
            disable-tunnel: [w87 _] -> w80
            frame Disabled {
              n25 = call "IMAQ Clear Overlay"("Image"=w88) -> ("error out"=w87:errorcluster)  [unwired: 9 in, 1 out]
            }
            frame Enabled {
            }
          }
          n26 = property on="Image" class="ImageControl"(error in=w80) -> ("ROI"=w79:T6)  [unwired: 1 in, 2 out]
          n27 = Unbundle By Name(w79) -> ("Global Rectangle"=w78:i32[])
          n28 = call "IMAQ ImageToArray"("Optional Rectangle"=w78, "Image"=w71) -> ("Image Pixels (U8)"=w77:u8[][])  [unwired: 2 in, 4 out]
          n29 = call "Sub_temp_data_maping.vi"("temp_data"=w77) -> ("mapping_temp"=w67:dbl[][])  [unwired: 10 in]
          n30 = Transpose 2D Array(2D array=w67) -> (transposed array=w73:dbl[][])
          n31 = Index Array(array=w73, index (col) #1=0 ("비활성화된 인덱스 (열)"), index (col) #2=1 ("비활성화된 인덱스 (열)")) -> (element #1=w70:dbl[], element #2=w69:dbl[])  [unwired: 2 in]
          n32 = Build Array(w69, w70) -> (→"강도 그래프 2":dbl[][])
          n33 = Build Array (concatenate)(w70, w69) -> (w68:dbl[])
          n34 = Unbundle By Name(w82) -> ("status"=w81:bool)
          n35 = local read "정지"() -> (w72:bool)
          n36 = call-poly <vilib>:"Mean.vi"("X"=w68) -> ("mean"=→"Heater temp 2":dbl)  [unwired: 1 out]
          n37 = Or(x=w81, y=w72) -> (x .or. y?=w66:bool)
        }
        n38 = call <vilib>:"IMAQdx Close Camera.vi"("error in"=w59, "Session In"=w62) -> ("error out"=→"error out":errorcluster)  [unwired: 9 in]
      }
      n39 = disable-structure shown="비활성화" {
        disable-tunnel: w49 -> [w89 _]
        frame Disabled {
          n40 = call "IMAQ Dispose"("Image"=w89) -> ()  [unwired: 5 in, 1 out]
        }
        frame Enabled {
        }
      }
    }
  }
  n41 = flat-sequence {
    tunnel: [w90] -> w10
    frame #0 {
      w90 = FALSE ("정지")
      n42 = local write "정지"(w90) -> ()
    }
  }
  n43 = Obtain Queue(name (unnamed)="strain" ("이름(이름없음)"), element data type=w1) -> (queue out=w8:refnum<queue>, error out=w6:errorcluster)  [unwired: 3 in, 1 out]
  n44 = while {
    tunnel: w4 -> [w111]
    tunnel: w3 -> [w110]
    tunnel: [w109] -> w14
    tunnel: [w108] -> w13
    tunnel: w10 -> [_]
    tunnel: w8 -> [w105]
    tunnel: [w104] -> w7
    tunnel: w6 -> [w103]
    tunnel: [w102] -> w5
    shift-right: [w97] -> _
    shift-left: _ -> [w98]
    i -> [w100]
    stop <- "정지" stop-if-true
    n45 = call-poly <vilib>:"DAQmx Read.vi"("task/channels in"=w110, "number of samples per channel"=100, "error in"=w111) -> ("task out"=w108:refnum<k21>, "data"=w94:waveform(dbl)[], "error out"=w109:errorcluster)  [unwired: 10 in]
    n46 = Tick Count (ms)() -> (millisecond timer value=w97:u32)
    n47 = call "strain-offset_fgv.vi"("열거형"=enum16{"write", "read"}."read") -> ("Strain_offset_data"=w92:waveform(dbl)[])  [unwired: 10 in]
    n48 = Subtract(1:w92, 2:w94) -> (0:w91:waveform(dbl)[])  [unwired: 1 in, 1 out]
    n49 = Bundle(cluster=cluster{"data":waveform(dbl)[], i32} {"data"=[], 0}, "data"=w91, w100) -> (w99:cluster{"data":waveform(dbl)[], i32})
    n50 = Subtract(x=w97, y=w98) -> (x-y=→"x-y 2":u32)
    n51 = case shown="참" "display" {
      tunnel: w91 -> [_ w112]
      frame False {
      }
      frame True {
        "Force raw graph" <- w112
        "Force raw chart" <- w112
      }
    }
    n52 = Enqueue Element(queue=w105, element=w99, error in (no error)=w103) -> (queue out=w104:refnum<queue>, error out=w102:errorcluster)  [unwired: 1 in, 1 out]
  }
  n53 = while {
    stop <- w113 stop-if-true
    n54 = event shown="[0] 타임아웃" {
      selector: _ -> [_ _ _]
      dyn-events: _ -> [_ _ _]
      timeout: _ -> [_ _ _]
      tunnel: [_ TRUE _] -> w113
      event Timeout {
        n55 = event-data() -> ()  [unwired: 1 in, 3 out]
      }
      event "정지": Value Change {
        n56 = event-data() -> ()  [unwired: 1 in, 6 out]
      }
      event "Force cal val": Value Change {
        n57 = event-data() -> ()  [unwired: 1 in, 6 out]
      }
    }
  }
  n58 = while {
    tunnel: w10 -> [_]
    shift-right: [w120] -> _
    shift-left: _ -> [w119]
    stop <- w121 stop-if-true
    n59 = call "DAQ 어시스턴트"() -> ("data"=w117:dynamicdata)  [unwired: 16 in, 3 out]
    "data" <- w117
    n60 = Tick Count (ms)() -> (millisecond timer value=w120:u32)
    n61 = Subtract(x=w120, y=w119) -> (x-y=→"x-y":u32)
    n62 = call "다이나믹 데이터로부터 변환"("Dynamic Data Type"=w117) -> ("Waveform"=w116:waveform(dbl))  [unwired: 3 in]
    n63 = local read "정지"() -> (w121:bool)
    n64 = local read "display"() -> (w115:bool)
    n65 = case shown="참" w115 {
      tunnel: w116 -> [_ w122]
      frame False {
      }
      frame True {
        "vaccum 차트 3" <- w122
        "vacum 2" <- w122
      }
    }
  }
  n66 = while {
    tunnel: w8 -> [w164]
    tunnel: w6 -> [w163]
    shift-right: [w155] -> _
    shift-left: _ -> [w154]
    i -> [w132]
    stop <- w162 stop-if-true
    n67 = disable-structure shown="비활성화" {
      disable-tunnel: [w169 _] -> w144
      disable-tunnel: [w167 _] -> w141
      disable-tunnel: [w166 _] -> w138
      disable-tunnel: [w165 _] -> w134
      frame Disabled {
        w165 = 0.4 ("trigger high check")
        (unwired) 0.3 ("y")
        (unwired) 0.3 ("y")
        (unwired) 0.3 ("y")
        w167 = 0.2 ("y")
        n68 = property on="Filtered force 차트" class="WFChart (엄격한)"() -> ("History Data"=w169:waveform(dbl)[][])  [unwired: 2 in, 2 out]
        n69 = Array Size(array=w169) -> (size(s)=w182:i32[])
        n70 = Array Size(array=w169) -> (size(s)=→"크기 2":i32[])
        n71 = Index Array(array=w182) -> (element=w181:i32)  [unwired: 1 in]
        n72 = Decrement(x=w181) -> (x-1=w180:i32)
        n73 = for {
          tunnel: w169 -> [w184] mode=indexing
          tunnel: [w183] -> w176 mode=indexing
          n74 = call "sub_minmaxmean.vi"("History Data"=w184) -> ("mean"=w183:dbl)  [unwired: 8 in, 2 out]
        }
        n75 = Index Array(array=w169, index (row) #2=w180) -> (element #1=w179:waveform(dbl)[], element #2=w178:waveform(dbl)[])  [unwired: 3 in]
        n76 = call "sub_minmaxmean.vi"("History Data"=w178) -> ("max"=w170:dbl)  [unwired: 8 in, 2 out]
        n77 = call "sub_minmaxmean.vi"("History Data"=w179) -> ("max"=w171:dbl)  [unwired: 8 in, 2 out]
        n78 = Array Max & Min(array=w176) -> (max value=w175:dbl)  [unwired: 3 out]
        n79 = Less?(x=w171, y=w167) -> (x < y?=w173:bool)
        n80 = Less?(x=w170, y=0.2) -> (x < y?=w172:bool)
        n81 = Greater?(x=w175, y=w165) -> (0:w174:bool)
        n82 = Compound Arithmetic op=AND(w174, w173, w172) -> (w166:bool)
      }
      frame Enabled {
      }
    }
    n83 = Dequeue Element(queue=w164, error in (no error)=w163) -> (element=w160:cluster{"data":waveform(dbl)[], i32}, error out=w162:errorcluster)  [unwired: 1 in, 2 out]
    n84 = Unbundle(w160) -> ("data"=w159:waveform(dbl)[])  [unwired: 1 out]
    n85 = call "필터"("Lower Cut-Off"="Lower Cut-Off", "Signal"=w159) -> ("Filtered Signal"=w158:dynamicdata)  [unwired: 8 in, 1 out]
    n86 = call "sub_dt.vi"() -> ("dt"=→"dt" →"웨이브폼 차트":u32)  [unwired: 11 in]
    n87 = call "다이나믹 데이터로부터 변환2"("Dynamic Data Type"=w158) -> ("Array of Waveform"=w157:waveform(dbl)[])  [unwired: 3 in]
    n88 = Multiply(x=w157, y=2246.0) -> (x*y=w145:waveform(dbl)[])
    "Filtered force 그래프" <- w145
    "Filtered force 차트" <- w145
    n89 = call "Strain-data-buffer.vi"("cmd"=enum16{"clear", "add", "read"}."add", "History Data"=w145) -> ("히스토리 데이터 out"=w140:waveform(dbl)[][])  [unwired: 9 in]
    n90 = Index Array(array=w145) -> (element #1=w131:waveform(dbl), element #2=w130:waveform(dbl), element #3=w129:waveform(dbl), element #4=w128:waveform(dbl))  [unwired: 4 in]
    n91 = call-poly <vilib>:"Basic Averaged DC-RMS.vi"("signal in"=w131) -> ("DC value"=w127:dbl)  [unwired: 7 in, 3 out]
    n92 = call-poly <vilib>:"Basic Averaged DC-RMS.vi"("signal in"=w130) -> ("DC value"=w126:dbl)  [unwired: 7 in, 3 out]
    n93 = call-poly <vilib>:"Basic Averaged DC-RMS.vi"("signal in"=w128) -> ("DC value"=w124:dbl)  [unwired: 7 in, 3 out]
    n94 = call-poly <vilib>:"Basic Averaged DC-RMS.vi"("signal in"=w129) -> ("DC value"=w125:dbl)  [unwired: 7 in, 3 out]
    n95 = Negate(x=w127) -> (-x=w135:dbl)
    n96 = Negate(x=w126) -> (-x=w136:dbl)
    n97 = local write "trigger"(w138) -> ()
    n98 = Add(x=w135, y=w125) -> (x+y=w153:dbl)
    n99 = Add(x=w136, y=w124) -> (x+y=w150:dbl)
    n100 = flat-sequence {
      tunnel: w134 -> [_]
      tunnel: w141 -> [_]
      tunnel: w140 -> [_]
      tunnel: [w187] -> w137
      frame #0 {
        n101 = call "sub_trigger-check.vi"("trigger low check"=0.2 ("y"), "trigger high check"="Force trigger minimum level") -> ("stop triiger"=w187:bool)  [unwired: 9 in]
        n102 = local write "triiger"(w187) -> ()
      }
    }
    n103 = Divide(x=w153, y=2.0) -> (x/y=w151:dbl)
    n104 = Divide(x=w150, y=2.0) -> (x/y=w149:dbl)
    n105 = Build Array(w151) -> (w143:dbl[])
    n106 = Build Array(w149) -> (w142:dbl[])
    n107 = Bundle(w142, w143) -> (→"XY 그래프":cluster{dbl[], dbl[]})  [unwired: 1 in]
    n108 = Select(t=w137, s=TRUE, f=w138) -> (s? t:f=w133:bool)
    n109 = case shown="참" w133 {
      selector: w133 -> [_ w224]
      tunnel: w144 -> [_ w192]
      tunnel: [w188 w222] -> w155
      tunnel: w154 -> [w188 w215]
      tunnel: w140 -> [_ _]
      tunnel: w137 -> [_ w189]
      frame False {
      }
      frame True {
        w237 = u16 1 items=["인덱스", "시간"] ("location mode")
        w236 = u16 0 items=["하강 에지", "상승 에지"] ("trigger slope")
        w238 = u16 1 items=["인덱스", "시간"] ("location mode")
        w239 = u16 1 items=["하강 에지", "상승 에지"] ("trigger slope")
        w203 = waveform(dbl) {"t0"=timestamp(0 s since 1904-01-01), "dt"=0.00062, "Y"=[]} ("원소")
        n110 = call "Strain-data-buffer.vi"("cmd"=enum16{"clear", "add", "read"}."read") -> ("히스토리 데이터 out"=w191:waveform(dbl)[][])  [unwired: 10 in]
        n111 = Select(t=w191, s=TRUE, f=w192) -> (s? t:f=w206:waveform(dbl)[][])
        n112 = local read "Heater temp 2"() -> (→"Heater temp":dbl)
        n113 = local read "vacum 2"() -> (→"vacum":dbl)
        n114 = case shown="참" "Force cal val" {
          tunnel: [w285 w290] -> w230
          tunnel: [w284 w289] -> w229
          tunnel: [w283 w288] -> w228
          tunnel: [w282 w287] -> w227
          frame False {
            n115 = local read "right mean 4"() -> (w282:dbl)
            n116 = local read "front mean"() -> (w285:dbl)
            n117 = local read "rear mean 3"() -> (w283:dbl)
            n118 = local read "left mean"() -> (w284:dbl)
          }
          frame True {
            (unwired) 0.31 ("y")
            (unwired) 0.39 ("y")
            (unwired) 0.64 ("y")
            (unwired) 0.29 ("y")
            n119 = property on="Strain rear" class="WFChart (엄격한)"() -> ("History Data"=w292:dbl[])  [unwired: 2 in, 2 out]
            n120 = property on="Strain left" class="WFChart (엄격한)"() -> ("History Data"=w291:dbl[])  [unwired: 2 in, 2 out]
            n121 = property on="Strain right" class="WFChart (엄격한)"() -> ("History Data"=w293:dbl[])  [unwired: 2 in, 2 out]
            n122 = property on="Strain front" class="WFChart (엄격한)"() -> ("History Data"=w294:dbl[])  [unwired: 2 in, 2 out]
            n123 = call-poly <vilib>:"Mean.vi"("X"=w294) -> ("mean"=w290:dbl)  [unwired: 1 out]
            n124 = call-poly <vilib>:"Mean.vi"("X"=w291) -> ("mean"=w289:dbl)  [unwired: 1 out]
            n125 = call-poly <vilib>:"Mean.vi"("X"=w292) -> ("mean"=w288:dbl)  [unwired: 1 out]
            n126 = call-poly <vilib>:"Mean.vi"("X"=w293) -> ("mean"=w287:dbl)  [unwired: 1 out]
            n127 = Bundle("mean"=w290, "mean"=w289, "mean"=w288, "mean"=w287) -> (→"strain high level mean":T4)  [unwired: 1 in]
          }
        }
        "front mean" <- w230
        "left mean" <- w229
        "rear mean 3" <- w228
        "right mean 4" <- w227
        n128 = for {
          tunnel: w206 -> [w309] mode=indexing
          shift-right: [w308] -> w204
          shift-left: w203 -> [w303]
          shift-right: [w307] -> w244
          shift-left: w203 -> [w302]
          shift-right: [w306] -> w245
          shift-left: w203 -> [w300]
          shift-right: [w305] -> w246
          shift-left: w203 -> [w297]
          n129 = Index Array(array=w309) -> (element #1=w304:waveform(dbl), element #2=w301:waveform(dbl), element #3=w299:waveform(dbl), element #4=w298:waveform(dbl))  [unwired: 4 in]
          n130 = call-poly <vilib>:"Append Waveforms.vi"("waveform B"=w304, "waveform A"=w303) -> ("waveform out"=w308:waveform(dbl))  [unwired: 8 in, 1 out]
          n131 = call-poly <vilib>:"Append Waveforms.vi"("waveform B"=w301, "waveform A"=w302) -> ("waveform out"=w307:waveform(dbl))  [unwired: 8 in, 1 out]
          n132 = call-poly <vilib>:"Append Waveforms.vi"("waveform B"=w299, "waveform A"=w300) -> ("waveform out"=w306:waveform(dbl))  [unwired: 8 in, 1 out]
          n133 = call-poly <vilib>:"Append Waveforms.vi"("waveform B"=w298, "waveform A"=w297) -> ("waveform out"=w305:waveform(dbl))  [unwired: 8 in, 1 out]
        }
        n134 = for {
          tunnel: w191 -> [w252] mode=indexing
          shift-right: [w264] -> w194
          shift-left: w203 -> [w259]
          shift-right: [w263] -> w197
          shift-left: w203 -> [w258]
          shift-right: [w262] -> w196
          shift-left: w203 -> [w256]
          shift-right: [w261] -> w195
          shift-left: w203 -> [w253]
          n135 = Index Array(array=w252) -> (element #1=w260:waveform(dbl), element #2=w257:waveform(dbl), element #3=w255:waveform(dbl), element #4=w254:waveform(dbl))  [unwired: 4 in]
          n136 = call-poly <vilib>:"Append Waveforms.vi"("waveform B"=w260, "waveform A"=w259) -> ("waveform out"=w264:waveform(dbl))  [unwired: 8 in, 1 out]
          n137 = call-poly <vilib>:"Append Waveforms.vi"("waveform B"=w257, "waveform A"=w258) -> ("waveform out"=w263:waveform(dbl))  [unwired: 8 in, 1 out]
          n138 = call-poly <vilib>:"Append Waveforms.vi"("waveform B"=w255, "waveform A"=w256) -> ("waveform out"=w262:waveform(dbl))  [unwired: 8 in, 1 out]
          n139 = call-poly <vilib>:"Append Waveforms.vi"("waveform B"=w254, "waveform A"=w253) -> ("waveform out"=w261:waveform(dbl))  [unwired: 8 in, 1 out]
        }
        n140 = Unbundle By Name(w194) -> ("Y"=w201:dbl[])
        n141 = Unbundle By Name(w197) -> ("Y"=w200:dbl[])
        n142 = Unbundle By Name(w196) -> ("Y"=w199:dbl[])
        n143 = Unbundle By Name(w195) -> ("Y"=w198:dbl[])
        n144 = call-poly <vilib>:"Amplitude and Levels.vi"("state settings"="state settings", "signal in"=w204) -> ("high state level"=w219:dbl)  [unwired: 6 in, 3 out]
        n145 = call-poly <vilib>:"Amplitude and Levels.vi"("state settings"="state settings", "signal in"=w244) -> ("high state level"=w217:dbl)  [unwired: 6 in, 3 out]
        n146 = call-poly <vilib>:"Amplitude and Levels.vi"("state settings"="state settings", "signal in"=w245) -> ("high state level"=w216:dbl)  [unwired: 6 in, 3 out]
        n147 = call-poly <vilib>:"Amplitude and Levels.vi"("state settings"="state settings", "signal in"=w246) -> ("high state level"=w221:dbl)  [unwired: 6 in, 3 out]
        n148 = Unbundle By Name(w204) -> ("Y"=w248:dbl[])
        n149 = Unbundle By Name(w244) -> ("Y"=w249:dbl[])
        n150 = Unbundle By Name(w245) -> ("Y"=w250:dbl[])
        n151 = Unbundle By Name(w246) -> ("Y"=w251:dbl[])
        n152 = Compound Arithmetic op=ADD(w201, w200, w199, w198) -> (w202:dbl[])
        n153 = First Call?() -> (First Call?: T/F=w214:bool)
        n154 = Compound Arithmetic op=ADD(w248, w249, w250, w251) -> (w247:dbl[])
        n155 = Or(x=w214, y="reset") -> ()  [unwired: 1 out]
        n156 = case shown="거짓" "reset" {
          tunnel: w221 -> [w268 w274]
          tunnel: [w268 w273] -> w220
          tunnel: w219 -> [w267 w280]
          tunnel: [w267 w279] -> w218
          tunnel: w217 -> [w266 w277]
          tunnel: [w266 w276] -> w211
          tunnel: w216 -> [w265 w275]
          tunnel: [w265 w278] -> w212
          tunnel: w215 -> [_ w281]
          frame False {
          }
          frame True {
            n157 = Unbundle(w281) -> ("high state level"=w269:dbl, "high state level"=w270:dbl, "high state level"=w271:dbl, "high state level"=w272:dbl)
            n158 = Subtract(x=w269, y=w280) -> (x-y=w279:dbl)
            n159 = Subtract(x=w270, y=w277) -> (x-y=w276:dbl)
            n160 = Subtract(x=w271, y=w275) -> (x-y=w278:dbl)
            n161 = Subtract(x=w272, y=w274) -> (x-y=w273:dbl)
          }
        }
        "level1" <- w218
        "level1 2" <- w211
        "level1 3" <- w212
        "level1 4" <- w220
        "Strain front" <- w218
        "Strain left" <- w211
        "Strain right" <- w220
        "Strain rear" <- w212
        "front" <- w218
        "rear" <- w212
        "left" <- w211
        "right" <- w220
        n162 = Bundle By Name(cluster=w194, "Y"=w202) -> (w190:waveform(dbl))
        "웨이브폼 그래프" <- w190
        n163 = Bundle By Name(cluster=w204, "Y"=w247) -> (w193:waveform(dbl))
        "Triggered Force graph" <- w193
        "웨이브폼 그래프 2" <- w193
        n164 = Bundle("high state level"=w218, "high state level"=w211, "high state level"=w212, "high state level"=w220) -> (w222:T7)  [unwired: 1 in]
        n165 = call-poly <vilib>:"Basic Level Trigger Detection.vi"("signal in"=w193, "level"="bonding time trigger edge level", "location mode"=w238, "trigger slope"=w239) -> ("trigger location"=w234:dbl)  [unwired: 9 in, 2 out]
        "trigger location" <- w234
        n166 = call-poly <vilib>:"Basic Level Trigger Detection.vi"("signal in"=w193, "level"="bonding time trigger edge level", "location mode"=w237, "trigger slope"=w236) -> ("trigger location"=w235:dbl)  [unwired: 9 in, 2 out]
        "trigger location 2" <- w235
        n167 = call-poly <vilib>:"Amplitude and Levels.vi"("state settings"="state settings", "signal in"=w193) -> ("high state level"=→"bonding force" →"웨이브폼 차트 2":dbl)  [unwired: 6 in, 3 out]
        n168 = Subtract(x=w235, y=w234) -> (x-y=→"Bondtime":dbl)
        n169 = Divide(x=w218, y=w230) -> (x/y=w243:dbl)
        n170 = Divide(x=w211, y=w229) -> (x/y=w242:dbl)
        n171 = flat-sequence {
          tunnel: w208 -> [_]
          tunnel: w190 -> [_]
          frame #0 {
            n172 = property on="Filtered force 차트" class="WFChart (엄격한)"("History Data"=waveform(dbl)[][] [[{"t0"=timestamp(0 s since 1904-01-01), "dt"=0.00062, "Y"=[]}]] ("히스토리 데이터")) -> ()  [unwired: 2 in, 2 out]
            n173 = call "Strain-data-buffer.vi"("cmd"=enum16{"clear", "add", "read"}."clear") -> ()  [unwired: 10 in, 1 out]
          }
        }
        n174 = Divide(x=w211, y=w228) -> (x/y=w240:dbl)
        n175 = Divide(x=w220, y=w227) -> (x/y=w241:dbl)
        n176 = call "Strain-data-buffer.vi"("cmd"=enum16{"clear", "add", "read"}."read") -> ("히스토리 데이터 out"=w208:waveform(dbl)[][])  [unwired: 10 in]
        n177 = Subtract(x=w218, y=w230) -> ()  [unwired: 1 out]
        n178 = Subtract(x=w211, y=w229) -> ()  [unwired: 1 out]
        n179 = Subtract(x=w211, y=w228) -> ()  [unwired: 1 out]
        n180 = Subtract(x=w220, y=w227) -> ()  [unwired: 1 out]
        n181 = Divide(x=w243, y=w242) -> ()  [unwired: 1 out]
        n182 = Divide(x=w240, y=w241) -> ()  [unwired: 1 out]
        "trigger" <- w224
        "triiger" <- w189
      }
    }
    "숫자형" <- w132
  }
  n183 = call <vilib>:"DAQmx Stop Task.vi"("task/channels in"=w13, "error in"=w14) -> ("task out"=w11:refnum<k21>, "error out"=w12:errorcluster)  [unwired: 12 in]
  n184 = Release Queue(queue=w7, error in (no error)=w5) -> ()  [unwired: 1 in, 3 out]
  n185 = call <vilib>:"DAQmx Clear Task.vi"("task in"=w11, "error in"=w12) -> ()  [unwired: 13 in, 1 out]
